vi "Embed Actor Core In Subpanel.vi"(8 "error in (no error)":errorcluster, 10 "Subpanel":refnum<vi>, 11 "AlbumImageActor in":refnum<class "AlbumImageActor.lvclass">) -> (0 "error out":errorcluster, 3 "AlbumImageActor out":refnum<class "AlbumImageActor.lvclass">)   [LabVIEW 2015, in "AlbumImageActor.lvlib" / "AlbumImageActor.lvclass"]
uses:
  AlbumImageActor.lvclass
  AlbumImageActor.lvclass/AlbumImageActor.ctl
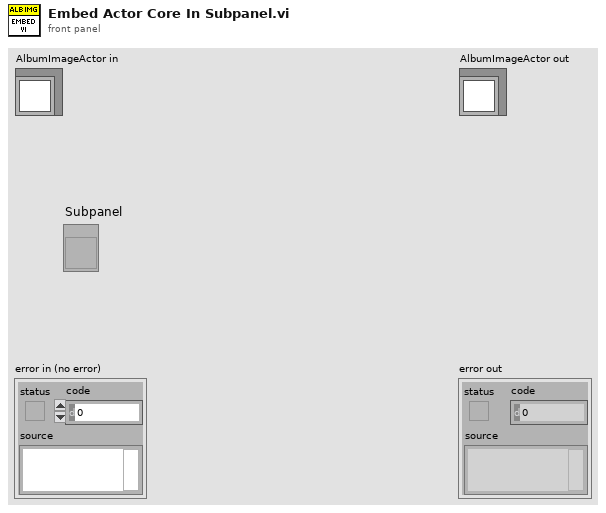
[diagram p1: front panel]
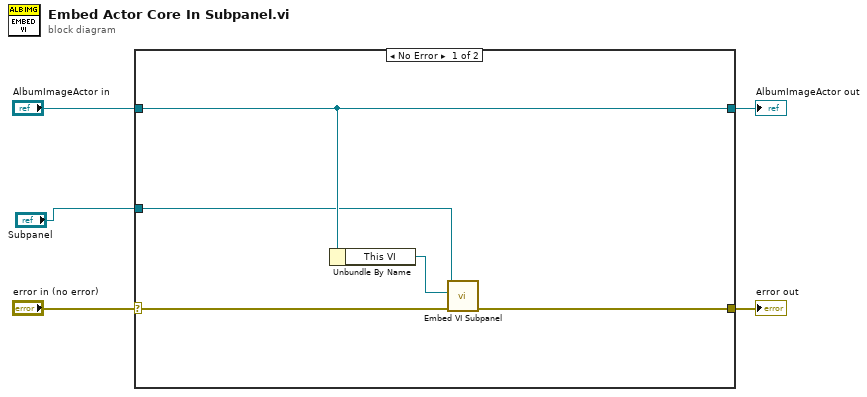
[diagram p0: block diagram]
diagram:
  n1 = case shown="No Error" "error in (no error)" {
    selector: "error in (no error)" -> [w9 w12]
    tunnel: [w6 w12] -> w4
    tunnel: [w8 w11] -> w2
    tunnel: "AlbumImageActor in" -> [w8 w11]
    tunnel: "Subpanel" -> [w7 _]
    frame No Error {
      n2 = Unbundle By Name(w8) -> ("This VI"=w10:refnum<vi>)
      n3 = call "Embed VI Subpanel.vi"("Error In"=w9, "VI Ref"=w10, "Subpanel Ref"=w7) -> ("Error Out"=w6:errorcluster)  [unwired: 8 in]
    }
    frame Error {
    }
  }
  "error out" <- w4
  "AlbumImageActor out" <- w2
